vi "globalSetUp.vi"(8 "error in":errorcluster, 11 "testcase-CSMSubModule in":refnum<class "testcase-CSMSubModule.lvclass">) -> (0 "error out":errorcluster, 3 "testcase-CSMSubModule out":refnum<class "testcase-CSMSubModule.lvclass">)   [LabVIEW 2017, in "testcase-CSMSubModule.lvclass"]
uses:
  testcase-CSMSubModule.lvclass
  <vilib>/addons/_JKI Toolkits/VI Tester/TestCase.llb/TestCase.lvclass
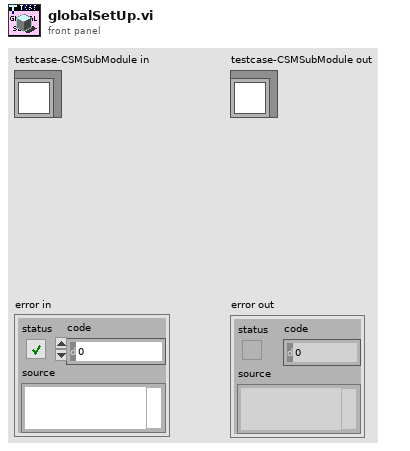
[diagram p1: front panel]
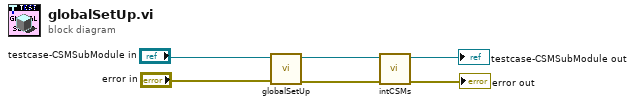
[diagram p0: block diagram]
diagram:
  n1 = call-parent "globalSetUp.vi"("error in (no error)"="error in", "TestCase in"="testcase-CSMSubModule in") -> ("error out"=w2:errorcluster, "TestCase out"=w5:refnum<class "testcase-CSMSubModule.lvclass">)  [unwired: 8 in]
  n2 = call "intCSMs.vi"("error in (no error)"=w2, "TestCase in"=w5) -> ("error out"=→"error out":errorcluster, "TestCase out"=→"testcase-CSMSubModule out":refnum<class "testcase-CSMSubModule.lvclass">)  [unwired: 8 in]
